vi "Get Instrument Type ID.vi"(8 "error in":errorcluster, 11 "instrument in":refnum<class "Instrument.lvclass">) -> (0 "error out":errorcluster, 2 "instrument type id":string, 3 "instrument out":refnum<class "Instrument.lvclass">)   [LabVIEW 2020, in "Keysight 34401A DMM Instrument.lvlib" / "Instrument.lvclass"]
uses:
  Instrument.lvclass
  Instrument.lvclass/Instrument.ctl
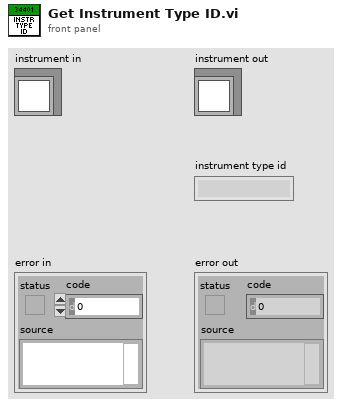
[diagram p1: front panel]
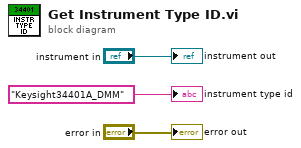
[diagram p0: block diagram]
diagram:
  "error out" <- "error in"
  "instrument out" <- "instrument in"
  "instrument type id" <- "Keysight34401A_DMM" ("instrument type id")
